vi "Get Sink References.vi"(8 "error in (no error)":errorcluster, 11 "Application Log in":refnum<class "Application Log.lvclass">) -> (0 "error out":errorcluster, 3 "Application Log out":refnum<class "Application Log.lvclass">, 5 "Sinks":refnum<data-value>[](array[refnum]), 7 "Names":string[](array[string]))   [LabVIEW 2016, in "Stream Log.lvlib" / "Application Log.lvclass"]
doc: "--\nCopyright © 2017 Composed SystemsI All rights reserved.\n\nAuthor: Jon McBee <jon.mcbee@composed.io>\n\nThis library is provided \"AS IS\" ,WITHOUT WARRANTIES OR\nCONDITIONS OF ANY KIND, either express or implied.\n\nComposed Systems -- composed.io\n\nStream 0.0.1.1\nJon McBee - Composed Systems\nCopyright (c) 2017, Composed Systems"
uses:
  <userlib>/Composed Systems/Stream/Log/Application Log/Application Log.lvclass
  <userlib>/Composed Systems/Stream/Log/Log Sink/Log Sink.lvclass
  <userlib>/Composed Systems/Stream/Log/Application Log/Application Log.lvclass/Application Log.ctl
  <userlib>/Composed Systems/Stream/Log/Sink Look Up Table/Sink Look Up Table.lvclass
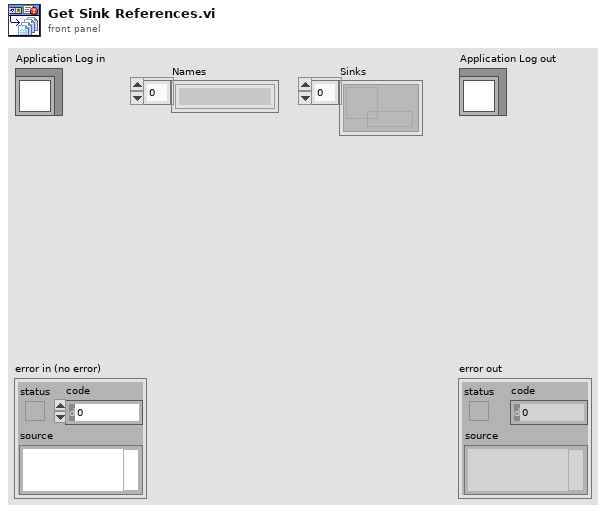
[diagram p1: front panel]
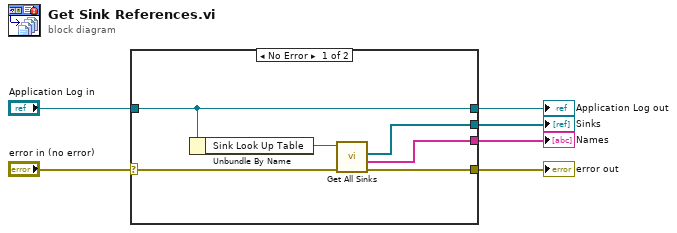
[diagram p0: block diagram]
diagram:
  n1 = case shown="No Error" "error in (no error)" {
    selector: "error in (no error)" -> [w10 w14]
    tunnel: [w9 w14] -> w5
    tunnel: [w11 w13] -> w3
    tunnel: "Application Log in" -> [w11 w13]
    tunnel: [w8 _] -> w2
    tunnel: [w7 _] -> w1
    frame No Error {
      n2 = Unbundle By Name(w11) -> ("Sink Look Up Table"=w12:refnum<class "Sink Look Up Table.lvclass">)
      n3 = call <userlib>:"Get All Sinks.vi"("error in (no error)"=w10, "Sink Look Up Table in"=w12) -> ("error out"=w9:errorcluster, "Names"=w7:string[], "Sinks"=w8:refnum<data-value>[])  [unwired: 6 in, 1 out]
    }
    frame Error {
    }
  }
  "error out" <- w5
  "Application Log out" <- w3
  "Sinks" <- w2
  "Names" <- w1
